vi "Test - Copy State From CSM to CSM 2.vi"() -> ()   [LabVIEW 2020]
uses:
  _csmHelper/CSM-Helper.lvclass/CSM-Helper.ctl
  _csmHelper/Properties/Read VI Ref.vi
  _csmHelper/API/Create From VI Reference.vi
  _csmHelper/API/Open Block Diagram.vi
  _csmHelper/Properties/Read States.vi
  _csmHelper/API/Start Undo.vi
  _csmHelper/API/Copy State.vi
  _csmHelper/API/Stop Undo.vi
  _csmHelper/API/Undo.vi
  _csmHelper/API/Destroy.vi
  _csmHelper/CSM-Helper.lvclass
panel:
  out "Array":T1(array[cluster])=[{"Idle", "error out"={"status"=FALSE, "code"=0, "source"=""}, "Execution:State"=enum."Idle"}, {"CSM Documentation", "error out"={"status"=FALSE, "code"=0, "source"=""}, "Execution:State"=enum."Idle"}, {"VI Reference", "error out"={"status"=FALSE, "code"=0, "source"=""}, "Execution:State"=enum."Bad"}, {"Error Handler", "error out"={"status"=TRUE, "code"=1055, "source"="Property Node in GObject Terminals.vi->CSM-Helper.lvclass:Diagram Connect Tunnel with Wire.vi->CSM-Helper.lvclass:Copy State.vi->Test - Copy State From CSM to CSM 2.vi"}, "Execution:State"=enum."Bad"}, {"Critical Error", "error out"={"status"=FALSE, "code"=0, "source"=""}, "Execution:State"=enum."Idle"}, {"Target Timeout Error", "error out"={"status"=FALSE, "code"=0, "source"=""}, "Execution:State"=enum."Idle"}, {"Target Error", "error out"={"status"=FALSE, "code"=0, "source"=""}, "Execution:State"=enum."Idle"}, {"Async Response", "error out"={"status"=FALSE, "code"=0, "source"=""}, "Execution:State"=enum."Bad"}, {"Response", "error out"={"status"=FALSE, "code"=0, "source"=""}, "Execution:State"=enum."Bad"}, {"Async Message Posted", "error out"={"status"=FALSE, "code"=0, "source"=""}, "Execution:State"=enum."Idle"}, {"Initialize Core Data", "error out"={"status"=FALSE, "code"=0, "source"=""}, "Execution:State"=enum."Idle"}, {"Exit", "error out"={"status"=FALSE, "code"=0, "source"=""}, "Execution:State"=enum."Idle"}, {"Data: Initialize", "error out"={"status"=FALSE, "code"=0, "source"=""}, "Execution:State"=enum."Idle"}, {"Data: Update Indicators", "error out"={"status"=FALSE, "code"=0, "source"=""}, "Execution:State"=enum."Idle"}, {"Data: Cleanup", "error out"={"status"=FALSE, "code"=0, "source"=""}, "Execution:State"=enum."Idle"}, {"Macro: Initialize", "error out"={"status"=FALSE, "code"=0, "source"=""}, "Execution:State"=enum."Idle"}, {"Macro: Exit", "error out"={"status"=FALSE, "code"=0, "source"=""}, "Execution:State"=enum."Idle"}, {"API: API1", "error out"={"status"=FALSE, "code"=0, "source"=""}, "Execution:State"=enum."Idle"}, {"API: API2", "error out"={"status"=FALSE, "code"=0, "source"=""}, "Execution:State"=enum."Idle"}, {"Action: action1", "error out"={"status"=FALSE, "code"=0, "source"=""}, "Execution:State"=enum."Idle"}, {"Action: action2", "error out"={"status"=FALSE, "code"=0, "source"=""}, "Execution:State"=enum."Idle"}]
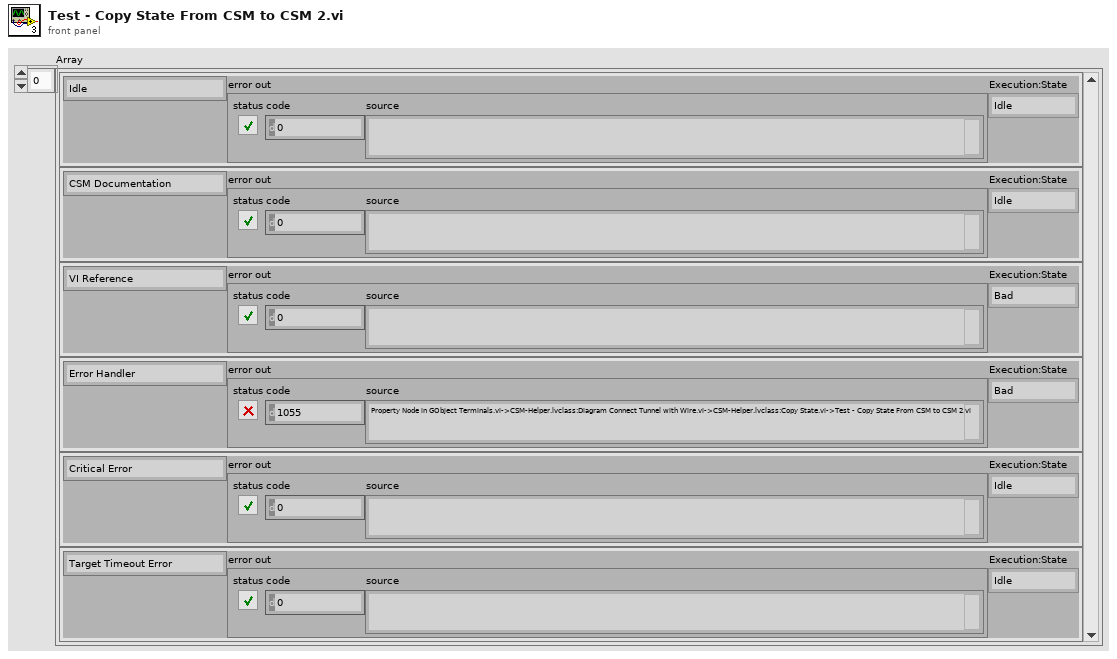
[diagram p1: front panel]
types:
  T1 = cluster{string, "error out":errorcluster, "Execution:State":enum32{"Bad", "Idle", "Run top level", "Running"}}[]
  T2 = enum32{"Bad", "Idle", "Run top level", "Running"}
  T3 = cluster{string, "error out":errorcluster, "Exec.State":enum32{"Bad", "Idle", "Run top level", "Running"}}
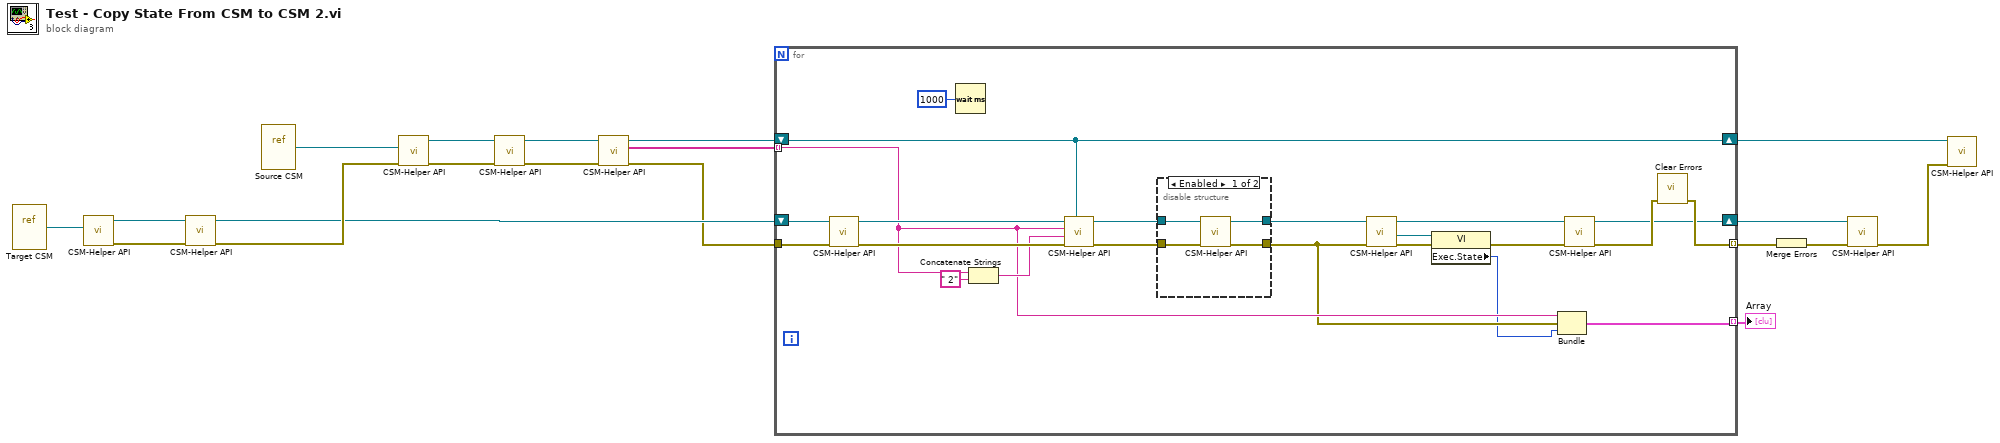
[diagram p0: block diagram]
diagram:
  n1 = vi-ref "Target CSM.vi"() -> (w18:refnum<vi>)
  n2 = call-poly "CSM-Helper API.vi"("VI"=w18) -> ("error out"=w15:errorcluster, "CSM-Helper.lvclass"=w14:refnum<class "CSM-Helper.lvclass">)  [unwired: 9 in]
  n3 = call-poly "CSM-Helper API.vi"("error in (no error)"=w15, "CSM-Helper in"=w14) -> ("error out"=w9:errorcluster, "CSM-Helper out"=w8:refnum<class "CSM-Helper.lvclass">)  [unwired: 8 in]
  n4 = vi-ref "Source CSM.vi"() -> (w19:refnum<vi>)
  n5 = call-poly "CSM-Helper API.vi"("error in (no error)"=w9, "VI"=w19) -> ("error out"=w12:errorcluster, "CSM-Helper.lvclass"=w13:refnum<class "CSM-Helper.lvclass">)  [unwired: 8 in]
  n6 = call-poly "CSM-Helper API.vi"("error in (no error)"=w12, "CSM-Helper in"=w13) -> ("error out"=w11:errorcluster, "CSM-Helper out"=w10:refnum<class "CSM-Helper.lvclass">)  [unwired: 8 in]
  n7 = call-poly "CSM-Helper API.vi"("error in (no error)"=w11, "CSM-Helper in"=w10) -> ("error out"=w7:errorcluster, "Value"=w3:string[], "CSM-Helper out"=w6:refnum<class "CSM-Helper.lvclass">)  [unwired: 7 in]
  n8 = for {
    shift-right: [w27] -> w17
    shift-left: w8 -> [w40]
    shift-right: [w35] -> w4
    shift-left: w6 -> [w35]
    tunnel: w3 -> [w31] mode=indexing
    tunnel: w7 -> [w39]
    tunnel: [w32] -> w16 mode=indexing
    tunnel: [w30] -> w1 mode=indexing
    n9 = call-poly "CSM-Helper API.vi"("error in (no error)"=w39, "CSM-Helper in"=w40) -> ("error out"=w38:errorcluster, "CSM-Helper out"=w37:refnum<class "CSM-Helper.lvclass">)  [unwired: 8 in]
    n10 = Wait (ms)(milliseconds to wait=u32 1000) -> ()  [unwired: 1 out]
    n11 = Concatenate Strings(w31, " 2" ("string")) -> (w34:string)
    n12 = call-poly "CSM-Helper API.vi"("SourceCSM"=w35, "error in (no error)"=w38, "New(Empty to Use same Name)"=w34, "Case"=w31, "CSM-Helper.lvclass"=w37) -> ("error out"=w36:errorcluster, "CSM-Helper out 2"=w41:refnum<class "CSM-Helper.lvclass">)  [unwired: 5 in]
    n13 = disable-structure shown="Enabled" {
      disable-tunnel: [w45 w47] -> w25
      disable-tunnel: w36 -> [w44 w46]
      disable-tunnel: [w43 w46] -> w26
      disable-tunnel: w41 -> [w42 w47]
      frame Enabled {
        n14 = call-poly "CSM-Helper API.vi"("error in (no error)"=w44, "CSM-Helper in"=w42) -> ("error out"=w43:errorcluster, "CSM-Helper out"=w45:refnum<class "CSM-Helper.lvclass">)  [unwired: 8 in]
      }
      frame Disabled {
      }
    }
    n15 = call-poly "CSM-Helper API.vi"("error in (no error)"=w26, "CSM-Helper in"=w25) -> ("error out"=w23:errorcluster, "VI"=w21:refnum<vi>, "CSM-Helper out"=w24:refnum<class "CSM-Helper.lvclass">)  [unwired: 7 in]
    n16 = property class="VI"(reference=w21, error in=w23) -> (error out=w22:errorcluster, "Exec.State"=w20:T2)  [unwired: 1 out]
    n17 = Bundle(w31, "error out"=w26, "Exec.State"=w20) -> (w30:T3)  [unwired: 1 in]
    n18 = call-poly "CSM-Helper API.vi"("error in (no error)"=w22, "CSM-Helper in"=w24) -> ("error out"=w28:errorcluster, "CSM-Helper out"=w27:refnum<class "CSM-Helper.lvclass">)  [unwired: 8 in]
    n19 = call <vilib>:"Clear Errors.vi"("error in (no error)"=w28) -> ("error out"=w32:errorcluster)  [unwired: 5 in, 1 out]
  }
  "Array" <- w1
  n20 = Merge Errors(w16) -> (w2:errorcluster)
  n21 = call-poly "CSM-Helper API.vi"("error in (no error)"=w2, "CSM-Helper in"=w17) -> ("error out"=w5:errorcluster)  [unwired: 8 in, 1 out]
  n22 = call-poly "CSM-Helper API.vi"("error in (no error)"=w5, "CSM-Helper in"=w4) -> ()  [unwired: 8 in, 2 out]
